vi "Dummy_Func_VAR_matTY.vi"(9 "Y":T1, 10 "T":dbl, 11 "Variant":variant) -> (0 "Error":bool, 3 "Output":T1)   [LabVIEW 2019]
uses:
  <vilib>/Analysis/Matrix/Datatypes/RealMatrix.ctl
  <vilib>/Analysis/Matrix/NI_Matrix.lvlib
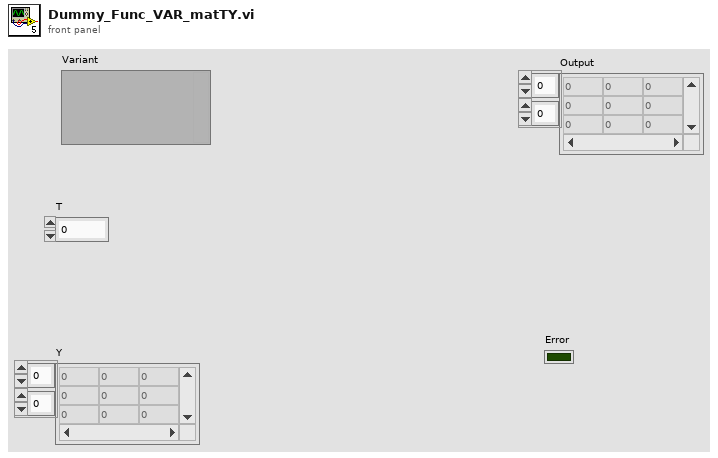
[diagram p1: front panel]
types:
  T1 = typedef "NI_Matrix.lvlib/RealMatrix.ctl" = dbl[][]
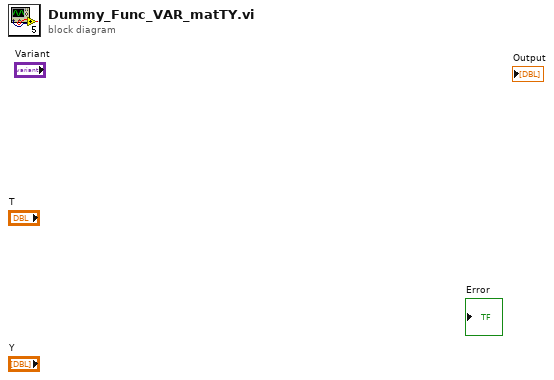
[diagram p0: block diagram]
diagram:
